vi "Add Filter.vi"(0 "Display State In":T1={"logTable"=refnum, "max items"=500, "displaydata"=[], "data"=[], "Auto Scroll"=TRUE, "current item"=500, "col headers"=[], "Add to Top"=TRUE, "Auto resize"=TRUE, "col size"=[], "filters"=[], "color cells"=[]}, 5 "column":string, 7 "filter":string[](array[string]), 9 "Container State":T3, 11 "error in (no error)":errorcluster) -> (4 "Display State Out":T1={"logTable"=refnum, "max items"=500, "displaydata"=[], "data"=[], "Auto Scroll"=TRUE, "current item"=500, "col headers"=[], "Add to Top"=TRUE, "Auto resize"=TRUE, "col size"=[], "filters"=[], "color cells"=[]}, 15 "error out":errorcluster)   [LabVIEW 2013, in "UI-DisplayTable(dev).xctl"]
uses:
  UI-DisplayTable(dev).xctl
  <vilib>/_xctls/Container State.ctl
  State.ctl
  Support/DEF-Filter.ctl
  <vilib>/_xctls/XControlSupport.lvlib
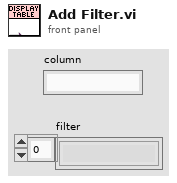
[diagram p1: front panel]
types:
  T1 = typedef "UI-DisplayTable(dev).xctl/State.ctl" = cluster{"logTable":refnum<vi>, "max items":i32, "displaydata":string[][], "data":string[][], "Auto Scroll":bool, "current item":i32, "col headers":string[], "Add to Top":bool, "Auto resize":bool, "col size":i32[], "filters":T2[], "color cells":cluster{"color cell":cluster{"Column":string, "Value":string, "Highlight Column":string}, "Color Box":u32}[]}
  T2 = typedef "UI-DisplayTable(dev).xctl/DEF-Filter.ctl" = cluster{"column":string, "value":string[]}
  T3 = typedef "XControlSupport.lvlib/Container State.ctl" = cluster{"Indicator?":bool, "Run Mode?":bool, " Refnum":refnum<vi>}
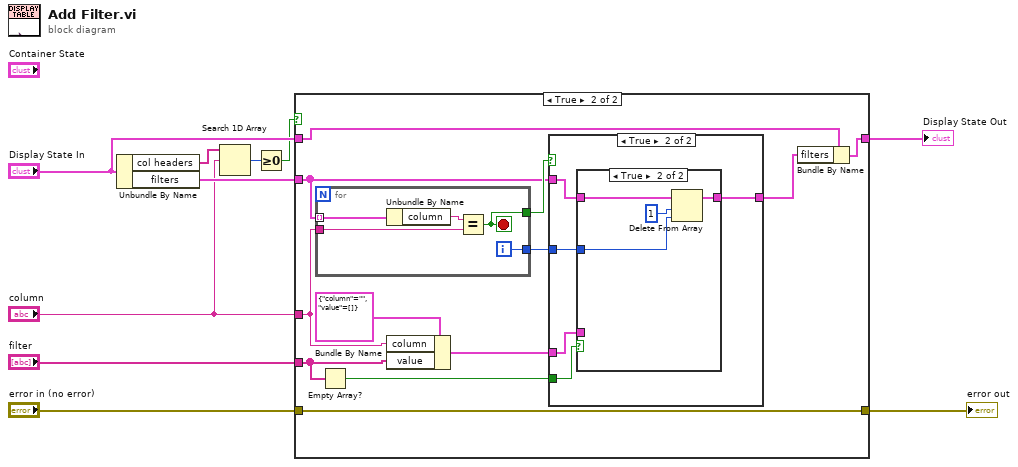
[diagram p0: block diagram]
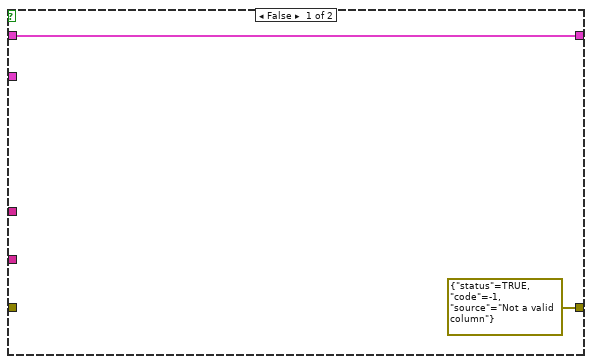
[diagram p2: hidden frame]
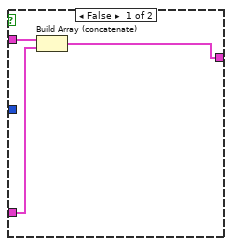
[diagram p3: hidden frame]
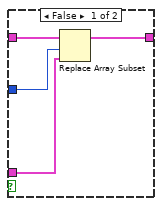
[diagram p4: hidden frame]
diagram:
  n1 = Unbundle By Name("Display State In") -> ("col headers"=w9:string[], "filters"=w10:T2[])
  n2 = Search 1D Array(1D array=w9, element="column") -> (index of element=w8:i32)  [unwired: 1 in]
  n3 = Greater Or Equal To 0?(x=w8) -> (x >= 0?=w1:bool)
  n4 = case shown="True" w1 {
    tunnel: w10 -> [_ w20]
    tunnel: "column" -> [_ w16]
    tunnel: "Display State In" -> [w12 w24]
    tunnel: [w12 w23] -> w3
    tunnel: "error in (no error)" -> [_ w22]
    tunnel: [errorcluster {"status"=TRUE, "code"=-1, "source"="Not a valid column"} ("error in (no error)") w22] -> w6
    tunnel: "filter" -> [_ w14]
    frame False {
    }
    frame True {
      n5 = for {
        tunnel: w20 -> [w43] mode=indexing
        tunnel: w16 -> [w44]
        tunnel: [w42] -> w18
        tunnel: [w41] -> w21
        i -> [w42]
        stop <- w41 stop-if-true
        n6 = Unbundle By Name(w43) -> ("column"=w45:string)
        n7 = Equal?(x=w45, y=w44) -> (x = y?=w41:bool)
      }
      n8 = Empty Array?(array=w14) -> (empty?=w13:bool)
      n9 = Bundle By Name(cluster=T2 {"column"="", "value"=[]} ("filter"), "column"=w16, "value"=w14) -> (w15:T2)
      n10 = case shown="True" w21 {
        tunnel: w20 -> [w27 w32]
        tunnel: [w26 w29] -> w19
        tunnel: w18 -> [_ w31]
        tunnel: w15 -> [w25 w30]
        tunnel: w13 -> [_ w28]
        frame False {
          n11 = Build Array (concatenate)(w27, w25) -> (w26:T2[])
        }
        frame True {
          n12 = case shown="True" w28 {
            tunnel: w32 -> [w36 w40]
            tunnel: w31 -> [w35 w38]
            tunnel: w30 -> [w34 _]
            tunnel: [w33 w39] -> w29
            frame False {
              n13 = Replace Array Subset(array=w36, new element=w34, index=w35) -> (w33:T2[])
            }
            frame True {
              n14 = Delete From Array(array=w40, length=1, index=w38) -> (array with subset deleted=w39:T2[])  [unwired: 1 out]
            }
          }
        }
      }
      n15 = Bundle By Name(cluster=w24, "filters"=w19) -> (w23:T1)
    }
  }
  "Display State Out" <- w3
  "error out" <- w6
